vi "Name Generator.vi"(7 "Keep Servo Error":bool, 10 "Group Specifier":string) -> (2 "Group Names":string[](array[string]))   [LabVIEW 2013]
uses:
  Source Group Type.ctl
  Space Group Type.ctl
  Cart Channel  Group Type.ctl
  Act Channel Group Type.ctl
panel:
  in  "Act Channel Group Type":T1
  in  "Cart Channel Group Type":T2
  in  "Space Group Type":T3
  in  "Source Group":T4
  # "Name formatting:\nSource/Space/Channels\nExternal sensors have no space or channels.\nConsolidated source has only cartesian space."
  # "Globbing recognize 3 special characters\n/ - is the delimiter between name tokens\n* - is a wildcard for all choices\n| - delimites a set of choices"
  # "Examples:\n/LBCB2/Act/* asks for all actuator groups for LBCB2\n/LBCB1/Cart/Cmd|Disp asks for the cartesian commands and\ndisplacements for LBCB1."
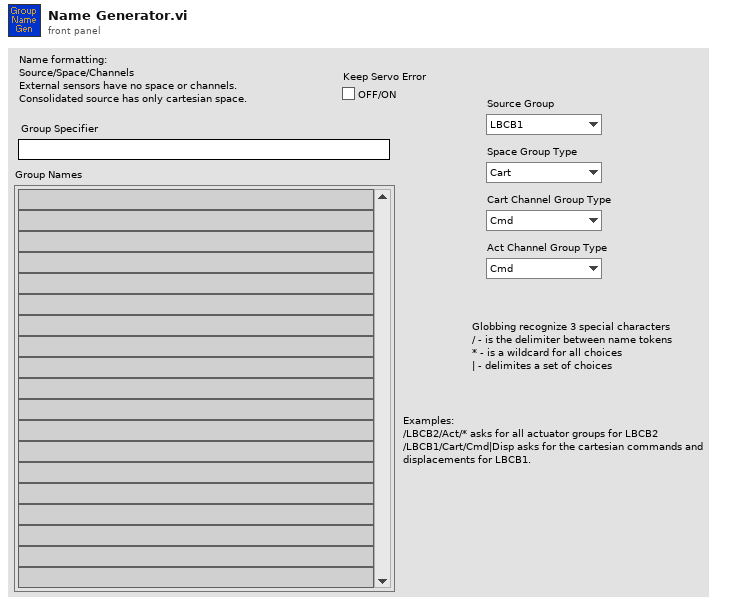
[diagram p1: front panel]
types:
  T1 = typedef "Act Channel Group Type.ctl" = enum16{"Cmd", "Disp", "Force", "ServoError"}
  T2 = typedef "Cart Channel  Group Type.ctl" = enum16{"Cmd", "Disp", "Load"}
  T3 = typedef "Space Group Type.ctl" = enum16{"Cart", "Act"}
  T4 = typedef "Source Group Type.ctl" = enum16{"LBCB1", "LBCB2", "Consolidated", "External"}
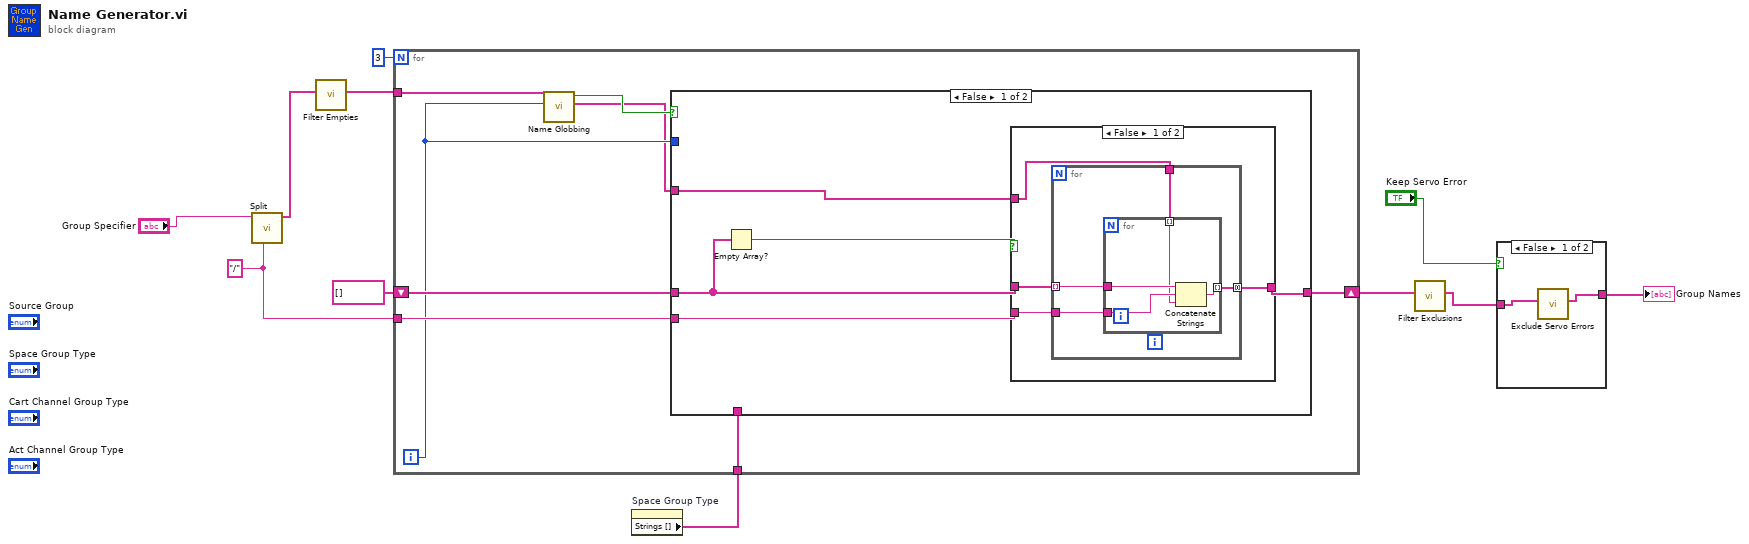
[diagram p0: block diagram]
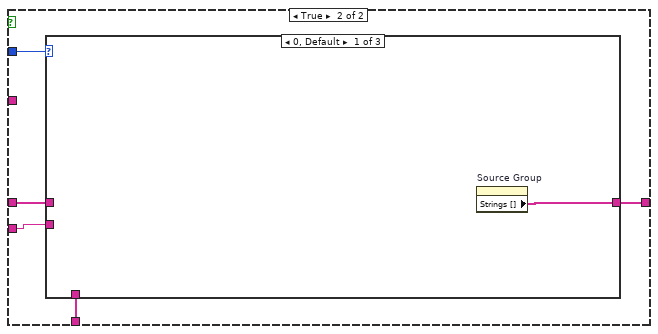
[diagram p4: hidden frame]
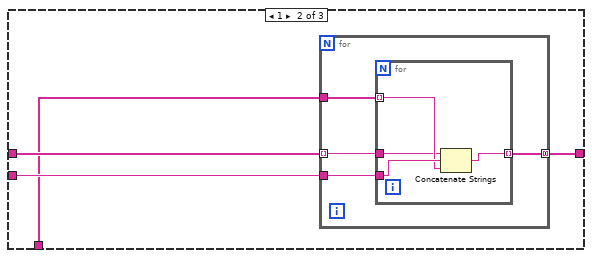
[diagram p5: hidden frame]
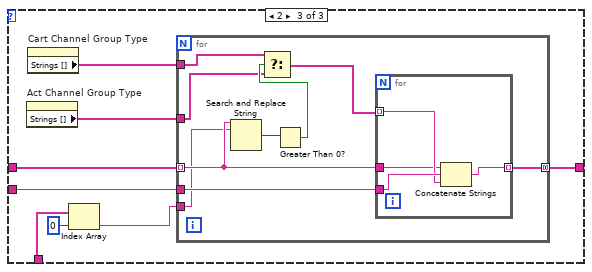
[diagram p6: hidden frame]
diagram:
  w10 = "/" ("delimiter")
  n1 = call "Split.vi"("delimiter"=w10, "String"="Group Specifier") -> ("Array Result"=w5:string[])  [unwired: 9 in]
  n2 = call "Filter Empties.vi"("In"=w5) -> ("Out"=w4:string[])  [unwired: 10 in]
  n3 = property on="Space Group Type" class="Enum (strict)"() -> ("Strings []"=w7:string[])  [unwired: 2 in, 2 out]
  n4 = for {
    N: 3 -> [_]
    tunnel: w4 -> [w14]
    shift-right: [w18] -> w8
    shift-left: string[] [] ("Strings []") -> [w17]
    tunnel: w10 -> [w16]
    tunnel: w7 -> [w15]
    i -> [w13]
    n5 = call "Name Globbing.vi"("Index"=w13, "Tokens"=w14) -> ("Selected Tokens"=w12:string[], "WildCard?"=w19:bool)  [unwired: 8 in]
    n6 = case shown="False" w19 {
      tunnel: w13 -> [_ w42]
      tunnel: [w21 w41] -> w18
      tunnel: w17 -> [w22 w40]
      tunnel: w12 -> [w24 _]
      tunnel: w16 -> [w20 w39]
      tunnel: w15 -> [_ w38]
      frame False {
        n7 = Empty Array?(array=w22) -> (empty?=w23:bool)
        n8 = case shown="False" w23 {
          tunnel: w22 -> [w28 _]
          tunnel: w24 -> [w26 w37]
          tunnel: [w25 w37] -> w21
          tunnel: w20 -> [w27 _]
          frame False {
            n9 = for {
              tunnel: w28 -> [w32] mode=indexing
              tunnel: w27 -> [w31]
              tunnel: w26 -> [w30]
              tunnel: [w29] -> w25 mode=concatenating
              n10 = for {
                tunnel: w32 -> [w36]
                tunnel: w31 -> [w35]
                tunnel: w30 -> [w34] mode=indexing
                tunnel: [w33] -> w29 mode=indexing
                n11 = Concatenate Strings(w36, w35, w34) -> (w33:string)
              }
            }
          }
          frame True {
          }
        }
      }
      frame True {
        n12 = case shown="0, Default" w42 {
          tunnel: [w43 w45 w61] -> w41
          tunnel: w40 -> [_ w47 w63]
          tunnel: w39 -> [_ w46 w62]
          tunnel: w38 -> [_ w44 w59]
          frame 0, Default {
            n13 = property on="Source Group" class="Enum (strict)"() -> ("Strings []"=w43:string[])  [unwired: 2 in, 2 out]
          }
          frame 1 {
            n14 = for {
              tunnel: w47 -> [w51] mode=indexing
              tunnel: w44 -> [w50]
              tunnel: w46 -> [w49]
              tunnel: [w48] -> w45 mode=concatenating
              n15 = for {
                tunnel: w51 -> [w53]
                tunnel: w50 -> [w54] mode=indexing
                tunnel: w49 -> [w55]
                tunnel: [w52] -> w48 mode=indexing
                n16 = Concatenate Strings(w53, w55, w54) -> (w52:string)
              }
            }
          }
          frame 2 {
            n17 = property on="Act Channel Group Type" class="Enum (strict)"() -> ("Strings []"=w56:string[])  [unwired: 2 in, 2 out]
            n18 = property on="Cart Channel Group Type" class="Enum (strict)"() -> ("Strings []"=w60:string[])  [unwired: 2 in, 2 out]
            n19 = Index Array(array=w59, index=0) -> (element=w57:string)
            n20 = for {
              tunnel: w63 -> [w69] mode=indexing
              tunnel: w60 -> [w65]
              tunnel: w62 -> [w72]
              tunnel: [w71] -> w61 mode=concatenating
              tunnel: w57 -> [w68]
              tunnel: w56 -> [w64]
              n21 = Search and Replace String(input string=w69, search string=w68) -> (number of replacements=w67:i32)  [unwired: 6 in, 3 out]
              n22 = Greater Than 0?(x=w67) -> (x > 0?=w66:bool)
              n23 = Select(t=w65, s=w66, f=w64) -> (s? t:f=w70:string[])
              n24 = for {
                tunnel: w69 -> [w74]
                tunnel: w70 -> [w75] mode=indexing
                tunnel: w72 -> [w76]
                tunnel: [w73] -> w71 mode=indexing
                n25 = Concatenate Strings(w74, w76, w75) -> (w73:string)
              }
            }
          }
        }
      }
    }
  }
  n26 = call "Filter Exclusions.vi"("Group Names"=w8) -> ("Group Names Out"=w2:string[])  [unwired: 10 in]
  n27 = case shown="False" "Keep Servo Error" {
    tunnel: w2 -> [w78 w79]
    tunnel: [w77 w79] -> w1
    frame False {
      n28 = call "Exclude Servo Errors.vi"("Group Names"=w78) -> ("Group Names Out"=w77:string[])  [unwired: 10 in]
    }
    frame True {
    }
  }
  "Group Names" <- w1
